vi "macro_TrajectoryReadFile.vi"   [LabVIEW 2019, in "Trajectory_Library.lvlib"]
uses:
  Trajectory_Library.lvlib
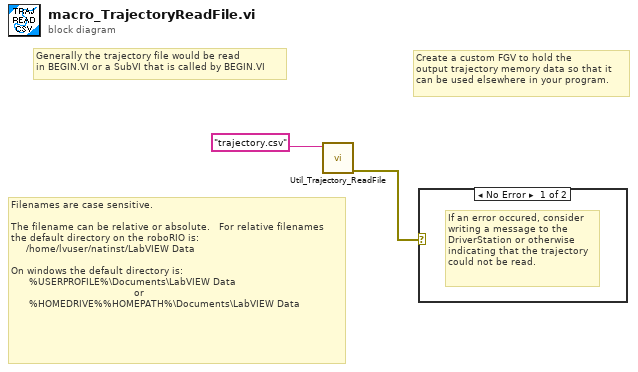
[diagram p0: block diagram]
diagram:
  # "Create a custom FGV to hold the \noutput trajectory memory data so that it\ncan be used elsewhere in your program."
  # "Generally the trajectory file would be read\nin BEGIN.VI or a SubVI that is called by BEGIN.VI"
  # "Filenames are case sensitive.\n\nThe filename can be relative or absolute.   For relative filenames\nthe default directory on the roboRIO is:\n     /home/lvuser/natinst/LabVIEW Data\n\nOn windows the default directory is:\n      %USERPROFILE%\\Documents\\LabVIEW Data\n                                         or\n      %HOMEDRIVE%%HOMEPATH%\\Documents\\LabVIEW Data"
  n1 = call "Util_Trajectory_ReadFile.vi"("FileName"="trajectory.csv") -> ("error out"=w1:errorcluster)  [unwired: 8 in, 2 out]
  n2 = case shown="No Error" w1 {
    frame No Error {
      # "If an error occured, consider\nwriting a message to the\nDriverStation or otherwise\nindicating that the trajectory\ncould not be read."
    }
    frame Error {
    }
  }
